vi "Dialog_Enter Wait Duration.vi"(8 "Error In":errorcluster) -> (0 "Error Out":errorcluster, 2 "Cancelled?":bool, 3 "Macro Command":string)   [LabVIEW 2012]
doc: "SciScan 1.2 160622\nThis VI has no controls.\nThis is a dummy whihc runs when user selects a macro command which does not require any arguments"
uses:
  Custom Controls and Typedefs/Macro_CommandStruct.ctl
  Custom Controls and Typedefs/Macro_Action_List.ctl
  Custom Controls and Typedefs/Macro_ArgumentStruct.ctl
panel:
  out "Macro Commands":T1
  in  "Cancel Button":bool
  in  "OK Button":bool
  in  "Seconds to Pause":dbl=1.0 min=1.0 step=1.0
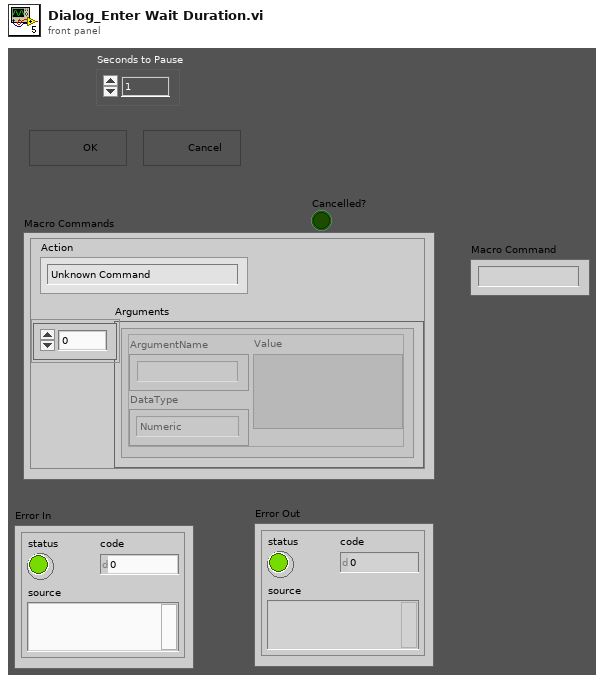
[diagram p1: front panel]
types:
  T1 = typedef "Macro_CommandStruct.ctl" = cluster{"Action":T2, "Arguments":T3[]}
  T2 = typedef "Macro_Action_List.ctl" = enum16{"Unknown Command", "2D.Frame.Scan", "2D.Line.Scan", "Load.Settings.File", "Move.To.Position", "Pause", "Z.Stack", "LOOP.Start", "LOOP.End", "Record", "Fast.Z", "Generic", "Slow.Z", "Tiling", "Preset.End"}
  T3 = typedef "Macro_ArgumentStruct.ctl" = cluster{"ArgumentName":string, "DataType":enum16{"Numeric", "String"}, "Value":variant}
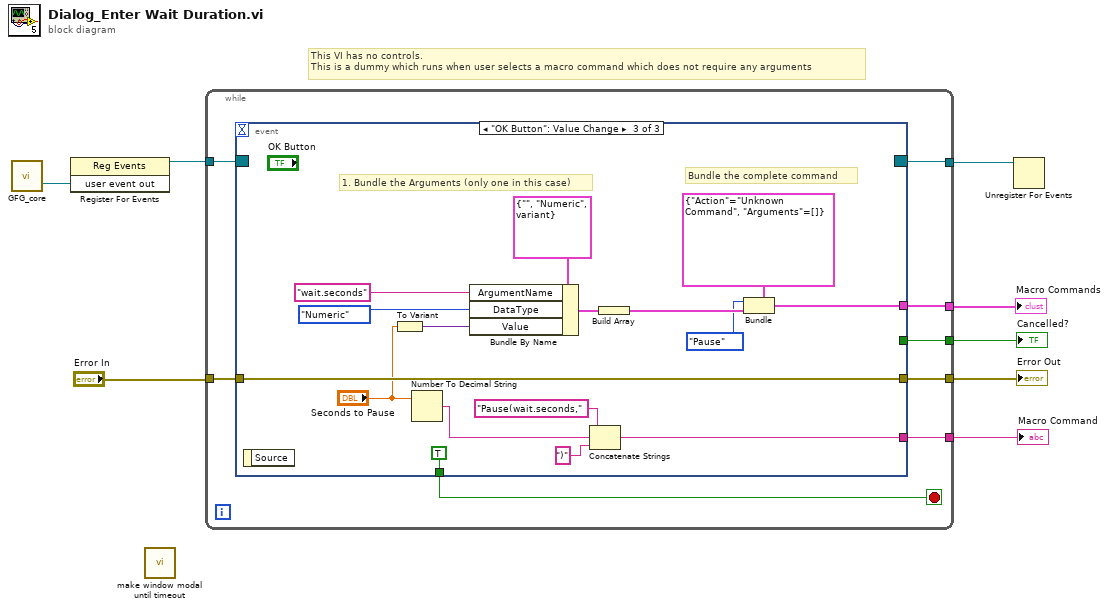
[diagram p0: block diagram]
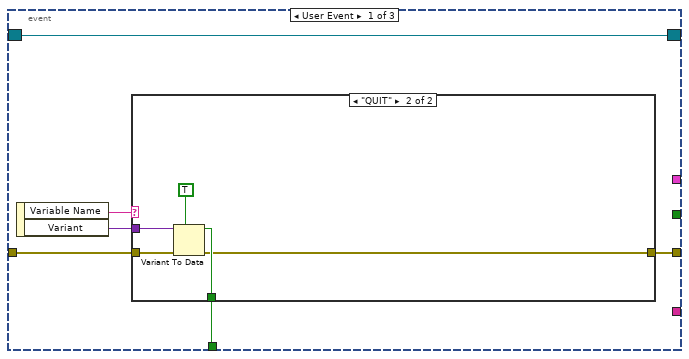
[diagram p2: hidden frame]
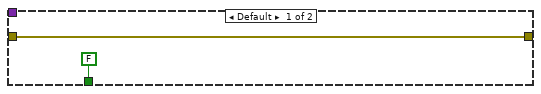
[diagram p3: hidden frame]
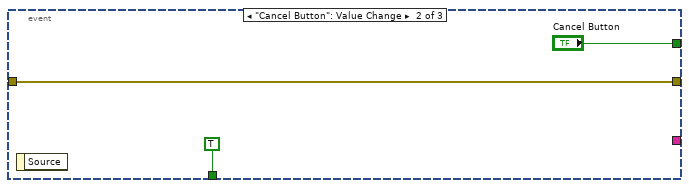
[diagram p4: hidden frame]
diagram:
  # "This VI has no controls.\nThis is a dummy which runs when user selects a macro command which does not require any arguments"
  n1 = call "GFG_core.vi"() -> ("user event out"=w8:refnum<user-event>)  [unwired: 13 in, 6 out]
  n2 = register-events(w8) -> (reference out=w7:refnum<event-registration>)  [unwired: 2 in, 1 out]
  n3 = call "make window modal until timeout.vi"() -> ()  [unwired: 12 in]
  n4 = while {
    tunnel: w7 -> [w16]
    tunnel: [w15] -> w6
    tunnel: "Error In" -> [w13]
    tunnel: [w12] -> w4
    tunnel: [w11] -> w3
    tunnel: [w10] -> w2
    tunnel: [w9] -> w1
    stop <- w14 stop-if-true
    n5 = event shown="[2] \"OK Button\": Value Change" {
      selector: w16 -> [w22 _ _]
      dyn-events: [w22 _ _] -> w15
      timeout: _ -> [_ _ _]
      tunnel: [w19 TRUE TRUE] -> w14
      tunnel: w13 -> [w18 w31 w39]
      tunnel: [w17 w31 w39] -> w12
      tunnel: [_ _ w40] -> w11
      tunnel: [_ "Cancel Button" _] -> w10
      tunnel: [_ _ w33] -> w9
      event User Event {
        n6 = event-data() -> ("Variable Name"=w21:string, "Variant"=w20:variant)  [unwired: 1 in]
        n7 = case shown="\"QUIT\"" w21 {
          tunnel: w20 -> [_ w28]
          tunnel: [FALSE w27] -> w19
          tunnel: w18 -> [w23 w26]
          tunnel: [w23 w25] -> w17
          frame Default {
          }
          frame "QUIT" {
            n8 = Variant To Data(error in=w26, type=TRUE, Variant=w28) -> (data=w27:bool, error out=w25:errorcluster)
          }
        }
      }
      event "Cancel Button": Value Change {
        n9 = event-data() -> ()  [unwired: 1 in, 1 out]
      }
      event "OK Button": Value Change {
        # "Bundle the complete command"
        # "1. Bundle the Arguments (only one in this case)"
        n10 = event-data() -> ()  [unwired: 1 in, 1 out]
        n11 = To Variant(anything="Seconds to Pause") -> (Variant=w45:variant)
        n12 = Number To Decimal String(number="Seconds to Pause") -> (decimal integer string=w35:string)  [unwired: 1 in]
        n13 = Bundle By Name(cluster=T3 {"ArgumentName"="", "DataType"=enum."Numeric", "Value"=variant} ("Arguments"), "ArgumentName"="wait.seconds", "DataType"=enum16{"Numeric", "String"}."Numeric", "Value"=w45) -> (w43:T3)
        n14 = Concatenate Strings("Pause(wait.seconds," ("ArgumentName"), w35, ")" ("string")) -> (w33:string)
        n15 = Build Array(w43) -> (w42:T3[])
        n16 = Bundle(cluster=T1 {"Action"=enum."Unknown Command", "Arguments"=[]} ("Macro Commands"), "Action"=Macro_Action_List."Pause", "Arguments"=w42) -> (w40:T1)
      }
    }
  }
  "Error Out" <- w4
  "Macro Commands" <- w3
  "Cancelled?" <- w2
  "Macro Command" <- w1
  n17 = Unregister For Events(event registration refnum=w6) -> ()  [unwired: 1 in, 1 out]
